vi "OpenCV CLAHE.vi"(6 "tileHeight":i32, 7 "tileWidth":i32, 8 "error in (no error)":errorcluster, 9 "ClipLimit":dbl, 10 "Image Dst":T1, 11 "Image Src":T1) -> (0 "error out":errorcluster, 1 "ClipLimit Out":dbl, 2 "Execution Time, ms":u32, 3 "Image Dst Out":T1, 4 "tileHeight Out":i32, 5 "tileWidth Out":i32)   [LabVIEW 2023]
uses:
  <vilib>/vision/Image Controls.llb/IMAQ Image.ctl
  build/OpenCVWrapper.dll
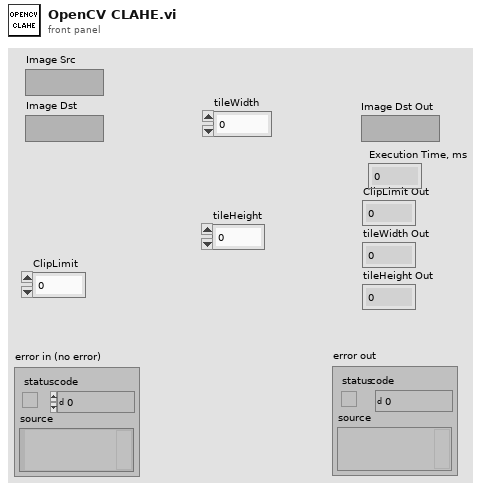
[diagram p1: front panel]
types:
  T1 = typedef "IMAQ Image.ctl" = refnum<image>
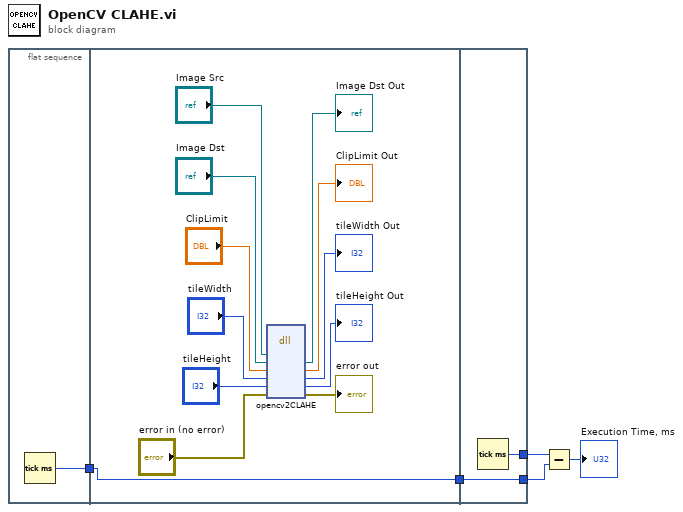
[diagram p0: block diagram]
diagram:
  n1 = flat-sequence {
    tunnel: [w6] -> w4
    tunnel: w4 -> [w7]
    tunnel: [w7] -> w3
    tunnel: [w20] -> w5
    tunnel: w3 -> [w19]
    tunnel: [w19] -> w2
    frame #0 {
      n2 = Tick Count (ms)() -> (millisecond timer value=w6:u32)
    }
    frame #1 {
      n3 = dll-call lib="D:/xe/OpenCVWrapper/build/OpenCVWrapper.dll" fn="opencv2CLAHE"("src"="Image Src", "dst"="Image Dst", "ClipLimit"="ClipLimit", "tileWidth"="tileWidth", "tileHeight"="tileHeight", "error"="error in (no error)") -> ("dst"=→"Image Dst Out":T1, "ClipLimit"=→"ClipLimit Out":dbl, "tileWidth"=→"tileWidth Out":i32, "tileHeight"=→"tileHeight Out":i32, "error"=→"error out":errorcluster)  [unwired: 5 in, 2 out]
    }
    frame #2 {
      n4 = Tick Count (ms)() -> (millisecond timer value=w20:u32)
    }
  }
  n5 = Subtract(x=w5, y=w2) -> (x-y=→"Execution Time, ms":u32)
